vi "Move Nested Items.vi"(8 "error in (no error)":errorcluster, 10 "Starting Top Position":i32, 11 "MenuButton in":refnum<class "MenuButton.lvclass">) -> (0 "error out":errorcluster, 2 "Ending Bottom Position":u32, 3 "MenuButton out":refnum<class "MenuButton.lvclass">)   [LabVIEW 2017, in "MenuButtons.lvlib" / "MenuButton.lvclass"]
uses:
  MenuButton.lvclass
  MenuButton.lvclass/MenuButton.ctl
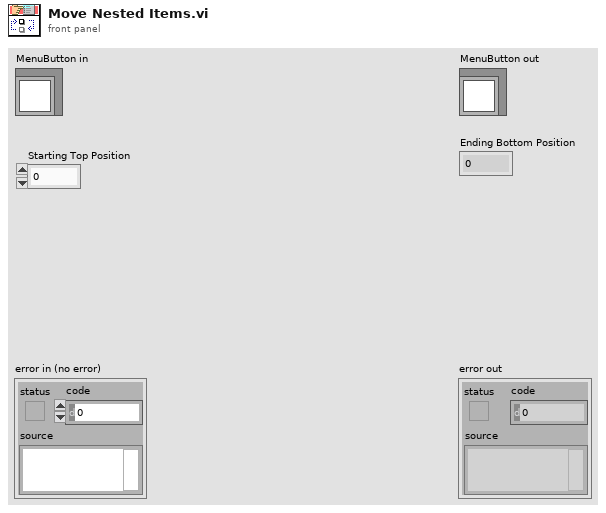
[diagram p1: front panel]
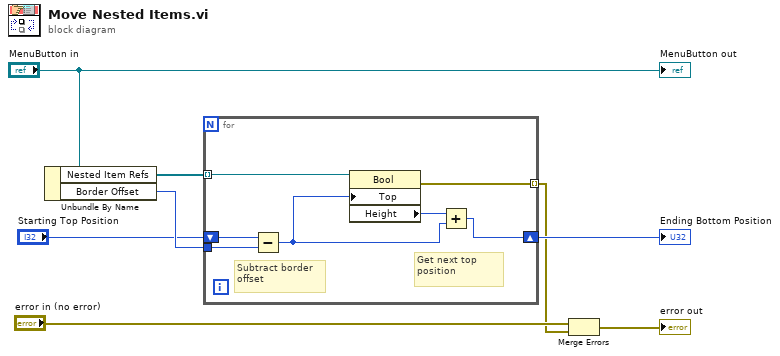
[diagram p0: block diagram]
diagram:
  n1 = Unbundle By Name("MenuButton in") -> ("Nested Item Refs"=w6:refnum<vi>[], "Border Offset"=w5:i32)
  n2 = for {
    tunnel: w6 -> [w15] mode=indexing
    tunnel: w5 -> [w13]
    shift-right: [w10] -> w3
    shift-left: "Starting Top Position" -> [w14]
    tunnel: [w9] -> w1 mode=indexing
    # "Get next top position"
    # "Subtract border offset"
    n3 = Subtract(x=w14, y=w13) -> (x-y=w11:u32)
    n4 = property class="Bool"(reference=w15, "Top"=w11) -> (error out=w9:errorcluster, "Height"=w12:u32)  [unwired: 1 in, 1 out]
    n5 = Add(x=w12, y=w11) -> (x+y=w10:u32)
  }
  "Ending Bottom Position" <- w3
  n6 = Merge Errors("error in (no error)", w1) -> (→"error out":errorcluster)
  "MenuButton out" <- "MenuButton in"
